vi "Send Ack--delete.vi"(8 "error in (no error)":errorcluster, 10 "Command Received":string, 11 "RemoteControl.ZMQ in":refnum<class "RemoteControl.ZMQ.lvclass">) -> (0 "error out":errorcluster, 3 "RemoteControl.ZMQ out":refnum<class "RemoteControl.ZMQ.lvclass">)   [LabVIEW 2019]
uses:
  RemoteControl.ZMQ.lvclass
  RemoteControl.ZMQ.lvclass/RemoteControl.ZMQ.ctl
  <vilib>/addons/zeromq/zmq_socket.lvclass
  C:/Users/patrick/Documents/GitHub/Instrument-Framework/lvsrc/SMOs/RemoteControl/RemoteControl.lvclass
  C:/Program Files (x86)/National Instruments/LabVIEW 2019/vi.lib/JKI/JKI SMO/SMO/SMO.lvclass
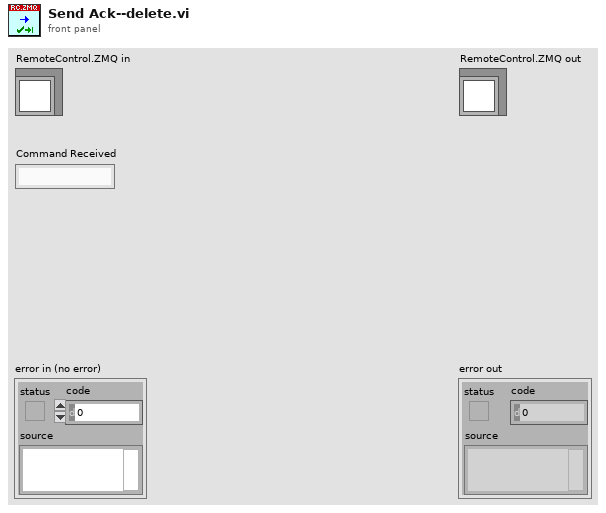
[diagram p1: front panel]
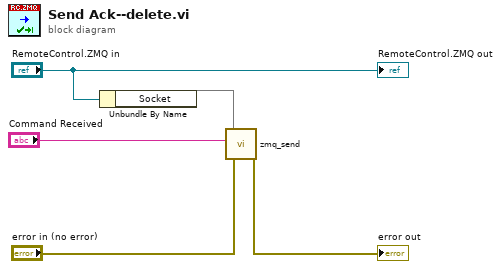
[diagram p0: block diagram]
diagram:
  n1 = Unbundle By Name("RemoteControl.ZMQ in") -> ("Socket"=w1)
  n2 = call <vilib>:"zmq_send.vi"("error in"="error in (no error)", "data"="Command Received", "socket in"=w1) -> ("error out"=→"error out":errorcluster)  [unwired: 4 in, 1 out]
  "RemoteControl.ZMQ out" <- "RemoteControl.ZMQ in"
